vi "GlobalGripper.vi"() -> ()   [LabVIEW 2020]
panel:
  in  "SEN_Piece_Held":enum16{"None", "Cube", "Cone"}(ring)
  # "DEVICE REFERENCE NAMES"
  # "CONSTANTS"
  # "DRIVER STATION DATA"
  # "SENSORS"
  # "OUTPUTS"
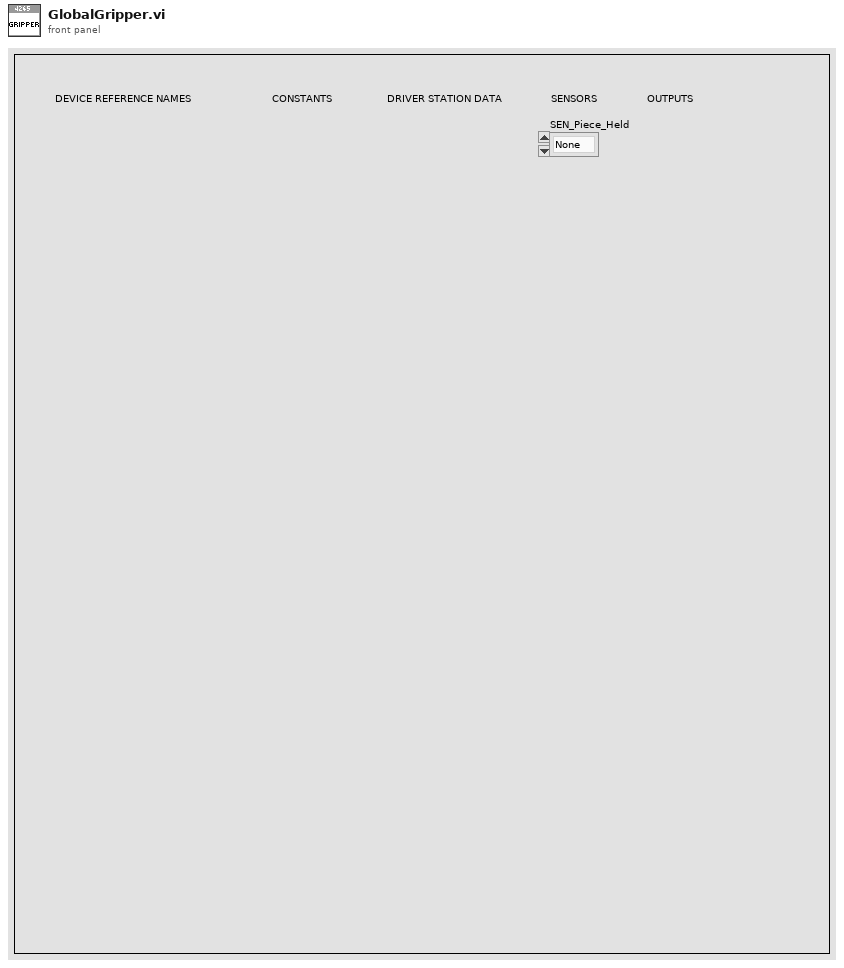
[diagram p1: front panel]
diagram:
